vi "Execute.vi"(8 "error in (no error)":errorcluster, 10 "System In":refnum<class "abs_System.lvclass">, 11 "Node in":refnum<class "Sequence.lvclass">) -> (0 "error out":errorcluster, 1 "Status":T1, 2 "System Out":refnum<class "abs_System.lvclass">, 3 "Node out":refnum<class "Sequence.lvclass">)   [LabVIEW 2021, in "BT.lvlib" / "Sequence.lvclass"]
uses:
  Sequence.lvclass
  C:/Users/Tim/Documents/LabVIEW/2021/Behaviour Tree/Source/abs_Composite/abs_Composite.lvclass
  abs_Node/Status.ctl
  abs_System/abs_System.lvclass
  abs_Composite/abs_Composite.lvclass/abs_Composite.ctl
  abs_Composite/Properties/Read Index.vi
  abs_Composite/Properties/Read Num Nodes.vi
  abs_Composite/Properties/Write Index.vi
  abs_Composite/abs_Composite.lvclass
  abs_Node/abs_Node.lvclass
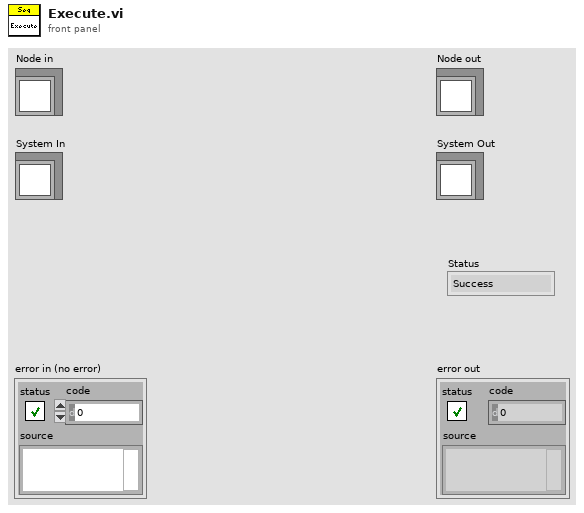
[diagram p1: front panel]
types:
  T1 = typedef "BT.lvlib/abs_Node.lvclass/Status.ctl" = enum16{"Success", "Failure", "Running"}
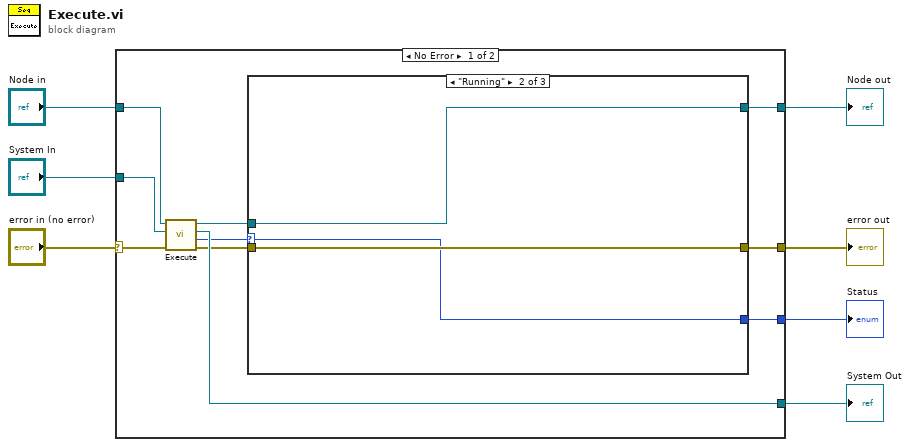
[diagram p0: block diagram]
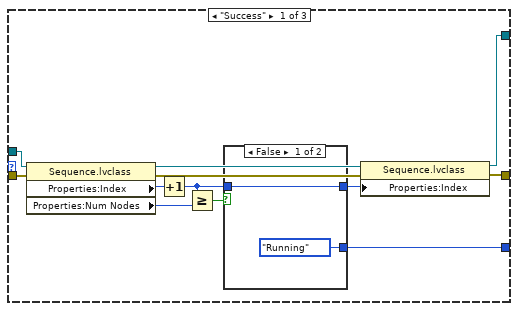
[diagram p2: hidden frame]
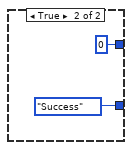
[diagram p3: hidden frame]
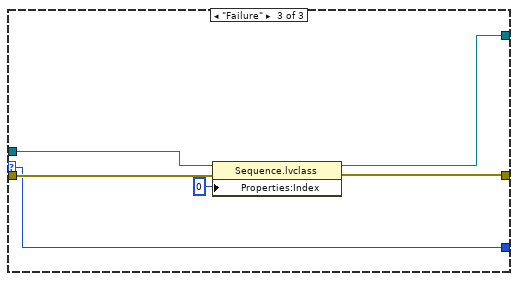
[diagram p4: hidden frame]
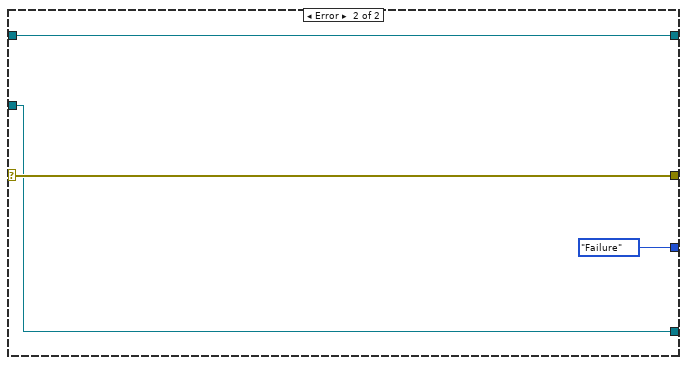
[diagram p5: hidden frame]
diagram:
  n1 = case shown="No Error" "error in (no error)" {
    selector: "error in (no error)" -> [w16 w45]
    tunnel: [w17 w44] -> w7
    tunnel: "System In" -> [w15 w44]
    tunnel: "Node in" -> [w14 w46]
    tunnel: [w12 w45] -> w3
    tunnel: [w9 w46] -> w2
    tunnel: [w8 Status."Failure" ("Status")] -> w1
    frame No Error {
      n2 = call-parent "Execute.vi"("error in (no error)"=w16, "System In"=w15, "Node in"=w14) -> ("error out"=w13:errorcluster, "Status"=w10:T1, "System Out"=w17:refnum<class "abs_System.lvclass">, "Node out"=w11:refnum<class "Sequence.lvclass">)  [unwired: 5 in]
      n3 = case shown="\"Running\"" w10 {
        selector: w10 -> [_ w34 w37]
        tunnel: w13 -> [w27 w35 w42]
        tunnel: [w29 w35 w41] -> w12
        tunnel: w11 -> [w25 w36 w40]
        tunnel: [w28 w36 w38] -> w9
        tunnel: [w18 w34 w37] -> w8
        frame "Success" {
          n4 = property class="Sequence.lvclass"(reference=w25, error in=w27) -> (reference out=w24:refnum<class "Sequence.lvclass">, error out=w26:errorcluster, "Properties:Index"=w23:i32, "Properties:Num Nodes"=w22:i32)
          n5 = Increment(x=w23) -> (x+1=w21:i32)
          n6 = Greater Or Equal?(x=w21, y=w22) -> (x >= y?=w19:bool)
          n7 = case shown="False" w19 {
            tunnel: w21 -> [w31 _]
            tunnel: [w31 0] -> w20
            tunnel: [Status."Running" ("Status") Status."Success" ("Status")] -> w18
            frame False {
            }
            frame True {
            }
          }
          n8 = property class="Sequence.lvclass"(reference=w24, error in=w26, "Properties:Index"=w20) -> (reference out=w28:refnum<class "Sequence.lvclass">, error out=w29:errorcluster)
        }
        frame "Running" {
        }
        frame "Failure" {
          n9 = property class="Sequence.lvclass"(reference=w40, error in=w42, "Properties:Index"=0 ("Index")) -> (reference out=w38:refnum<class "Sequence.lvclass">, error out=w41:errorcluster)
        }
      }
    }
    frame Error {
    }
  }
  "error out" <- w3
  "Node out" <- w2
  "Status" <- w1
  "System Out" <- w7
